vi "WPI_SwitchPublishInfo.vi"(10 "Name":string, 11 "SwitchDevRef":T1={"DevStatus"={"status"=FALSE, "code"=0, "source"=""}, "DIO Channel"=enum."Invalid", "CntIndex"=enum."Invalid", "Normally Closed"=FALSE}) -> ()   [LabVIEW 2017]
uses:
  <vilib>/Rock Robotics/WPI/Switch/WPI_SwitchDevRef.ctl
  <vilib>/Rock Robotics/SystemInterfaces/DIO/FPGA_DIOChannel.ctl
  <vilib>/Rock Robotics/SystemInterfaces/Counter/FPGA_CounterCtrSystemIndex.ctl
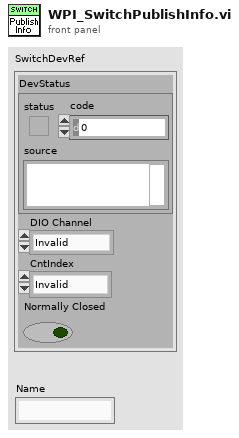
[diagram p1: front panel]
types:
  T1 = typedef "WPI_SwitchDevRef.ctl" = cluster{"DevStatus":errorcluster, "DIO Channel":T2, "CntIndex":T3, "Normally Closed":bool}
  T2 = typedef "FPGA_DIOChannel.ctl" = enum8{"DIO 0", "DIO 1", "DIO 2", "DIO 3", "DIO 4", "DIO 5", "DIO 6", "DIO 7", "DIO 8", "DIO 9", "DIO MXP 0", "DIO MXP 1", "DIO MXP 2", "DIO MXP 3", "DIO MXP 4", "DIO MXP 5", "DIO MXP 6", "DIO MXP 7", "DIO MXP 8", "DIO MXP 9", "DIO MXP 10", "DIO MXP 11", "DIO MXP 12", "DIO MXP 13", "DIO MXP 14", "DIO MXP 15", "SPI Port CS1", "SPI Port CS2", "SPI Port CS3", "SPI Port MISO", "SPI Port MOSI", "Invalid"}
  T3 = typedef "FPGA_CounterCtrSystemIndex.ctl" = enum8{"Ctr 0", "Ctr 1", "Ctr 2", "Ctr 3", "Ctr 4", "Ctr 5", "Ctr 6", "Ctr 7", "Invalid"}
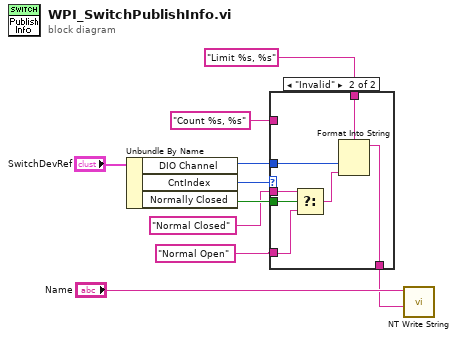
[diagram p0: block diagram]
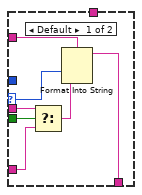
[diagram p2: hidden frame]
diagram:
  n1 = Unbundle By Name("SwitchDevRef") -> ("DIO Channel"=w10:T2, "CntIndex"=w5:T3, "Normally Closed"=w4:bool)
  n2 = case shown="\"Invalid\"" w5 {
    selector: w5 -> [w16 _]
    tunnel: w10 -> [_ w24]
    tunnel: [w11 w23] -> w8
    tunnel: "Limit %s, %s" ("format string") -> [_ w22]
    tunnel: w4 -> [w15 w21]
    tunnel: "Normal Open" ("format string") -> [w13 w20]
    tunnel: "Normal Closed" ("format string") -> [w14 w19]
    tunnel: "Count %s, %s" ("format string") -> [w17 _]
    frame Default {
      n3 = Select(t=w14, s=w15, f=w13) -> (s? t:f=w12:string)
      n4 = Format Into String(format string=w17, w16, w12) -> (resulting string=w11:string)  [unwired: 2 in, 1 out]
    }
    frame "Invalid" {
      n5 = Select(t=w19, s=w21, f=w20) -> (s? t:f=w18:string)
      n6 = Format Into String(format string=w22, w24, w18) -> (resulting string=w23:string)  [unwired: 2 in, 1 out]
    }
  }
  n7 = call <vilib>:"NT Write String.vi"("String"=w8, "Name"="Name") -> ()  [unwired: 9 in, 1 out]
